vi "String Parser.vi"() -> ()   [LabVIEW 2017]
uses:
  <vilib>/regexp/Match Regular Expression.xnode
panel:
  out "String":string
  out "Array":T1(array[cluster])
  out "text":string
  in  "Path":path
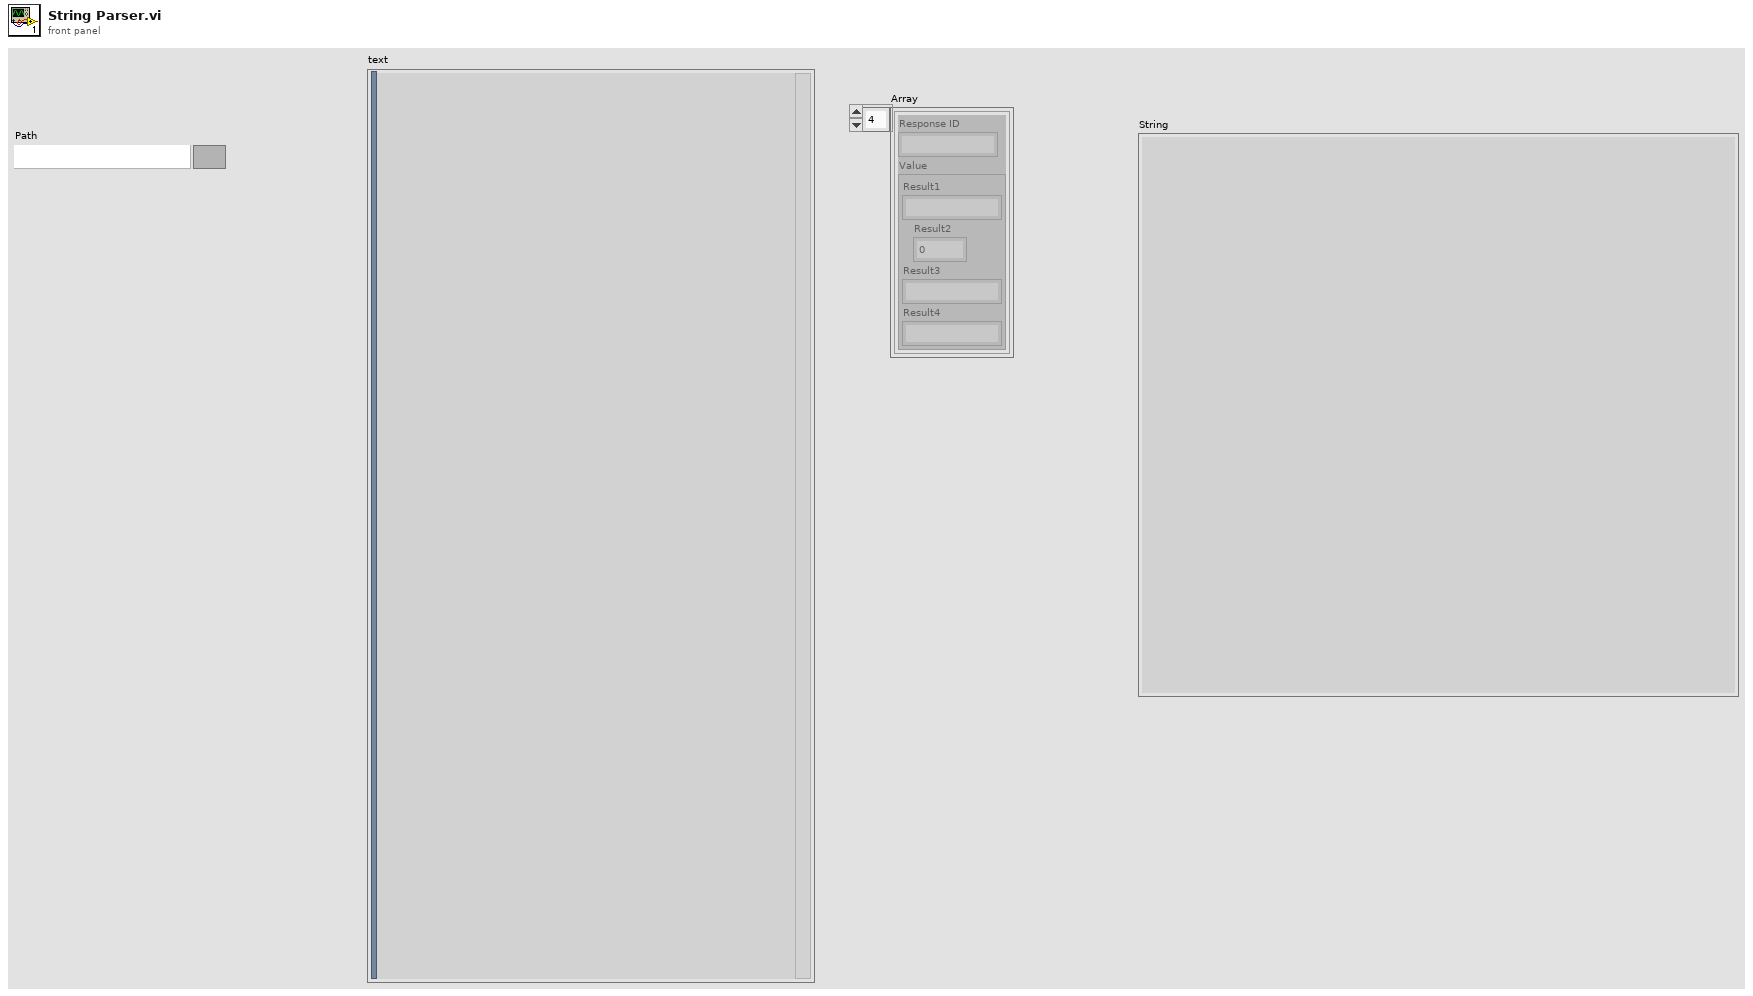
[diagram p1: front panel]
types:
  T1 = cluster{"Response ID":string, "Value":cluster{"Result1":string, "Result2":dbl, "Result3":string, "Result4":string}}[]
  T2 = cluster{"Response ID":string, "Value":cluster{"Result1":string, "Result2":dbl, "Result3":string, "Result4":string}}
  T3 = cluster{"Result1":string, "Result2":dbl, "Result3":string, "Result4":string}
  T4 = cluster{"Result1":string, "Result2":string, "Result3":string, "Result4":string}
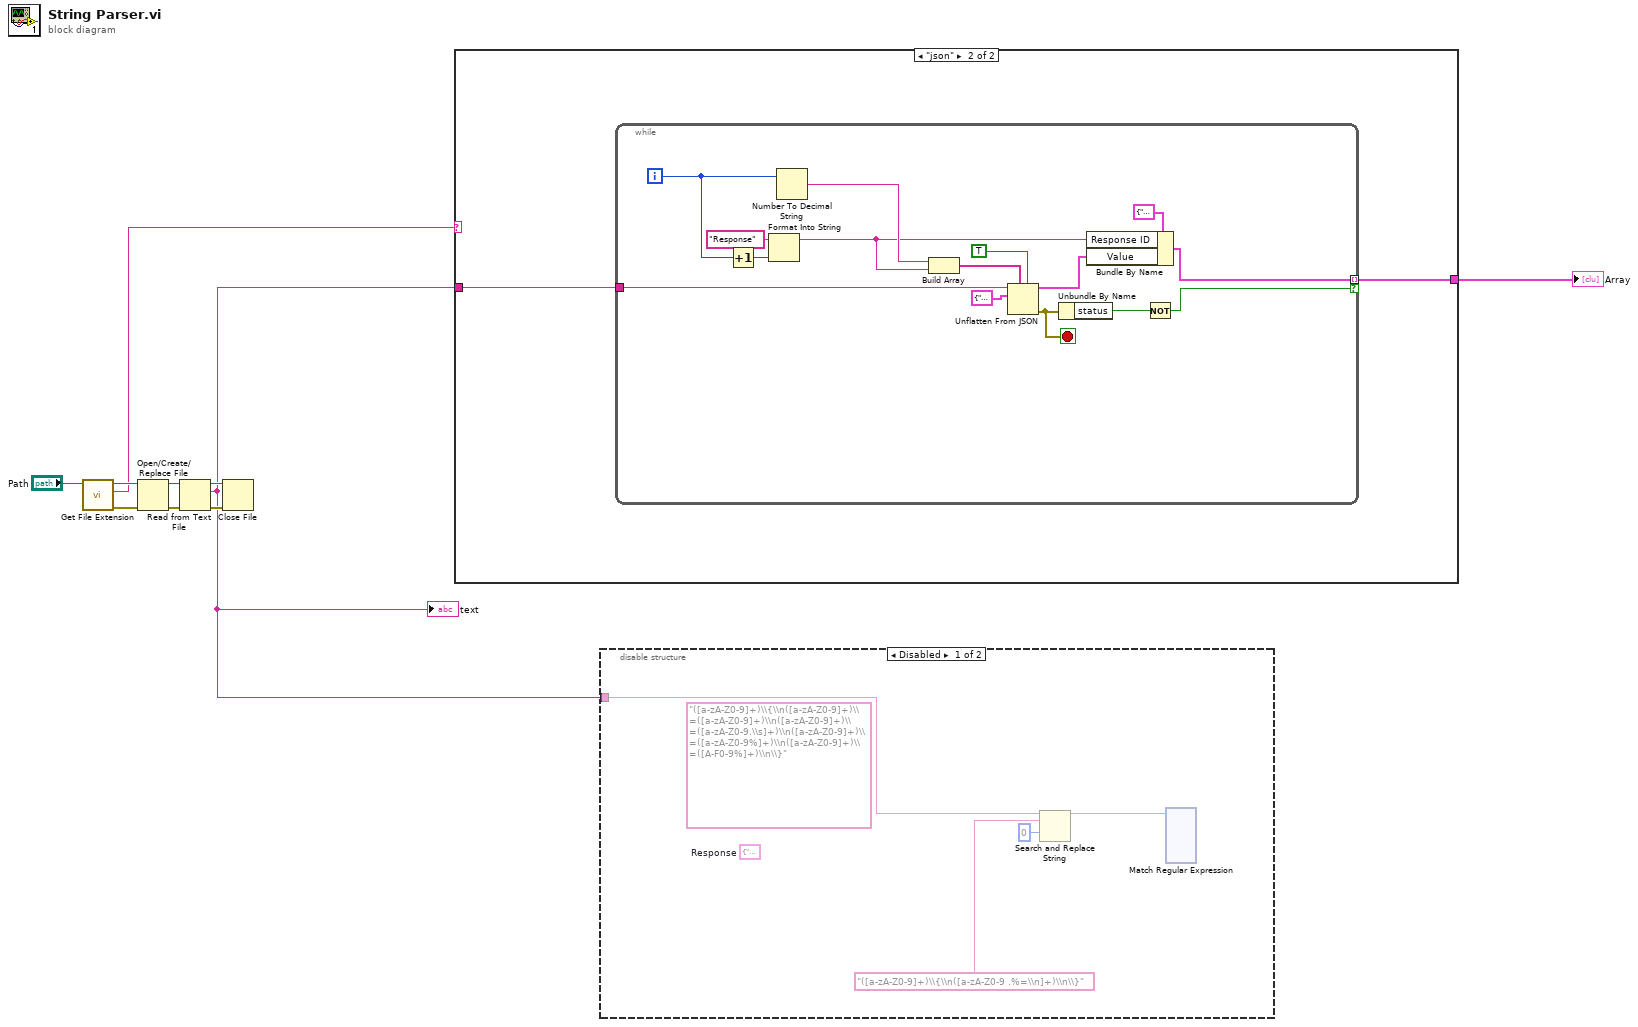
[diagram p0: block diagram]
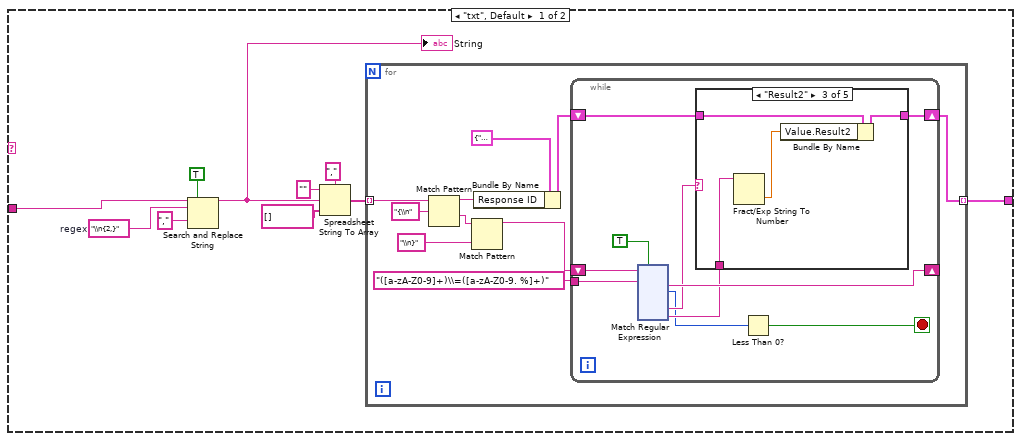
[diagram p2: hidden frame]
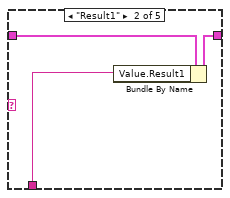
[diagram p4: hidden frame]
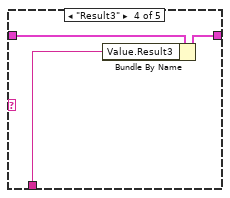
[diagram p5: hidden frame]
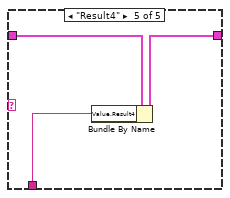
[diagram p6: hidden frame]
diagram:
  n1 = call <vilib>:"Get File Extension.vi"("file"="Path") -> ("error out"=w1:errorcluster, "lowercase file extension"=w4:string)  [unwired: 6 in, 3 out]
  n2 = Open/Create/Replace File(file path (use dialog)="Path", error in=w1) -> (refnum out=w9:refnum<file>, error out=w8:errorcluster)  [unwired: 4 in, 1 out]
  n3 = Read from Text File(file (use dialog)=w9, error in=w8) -> (refnum out=w7:refnum<file>, text=w2:string, error out=w6:errorcluster)  [unwired: 2 in, 1 out]
  "text" <- w2
  n4 = Close File(refnum=w7, error in=w6) -> ()  [unwired: 2 out]
  n5 = case shown="\"json\"" w4 {
    tunnel: w2 -> [w19 w172]
    tunnel: [w10 w171] -> w3
    frame "txt", Default {
      w18 = "\\n{2,}"  # regex
      n6 = Search and Replace String(replace all?=TRUE ("replace all? (F)"), input string=w19, search string=w18, replace string="," ("replace string (\"\")")) -> (result string=w12:string)  [unwired: 4 in, 3 out]
      "String" <- w12
      n7 = Spreadsheet String To Array(delimiter (Tab)=",", format string="", spreadsheet string=w12, array type (2D Dbl)=string[] [] ("spreadsheet string")) -> (array=w11:string[])
      n8 = for {
        tunnel: w11 -> [w29] mode=indexing
        tunnel: [w20] -> w10 mode=indexing
        n9 = Match Pattern(string=w29, regular expression="{\\n") -> (before substring=w27:string, after substring=w26:string)  [unwired: 1 in, 2 out]
        n10 = Match Pattern(string=w26, regular expression="\\n}") -> (before substring=w21:string)  [unwired: 1 in, 3 out]
        n11 = Bundle By Name(cluster=T2 {"Response ID"="", "Value"={"Result1"="", "Result2"=0.0, "Result3"="", "Result4"=""}}, "Response ID"=w27) -> (w23:T2)
        n12 = while {
          tunnel: "([a-zA-Z0-9]+)\\=([a-zA-Z0-9. %]+)" ("regular expression") -> [w38]
          shift-right: [w34] -> _
          shift-left: w21 -> [w37]
          shift-right: [w35] -> w20
          shift-left: w23 -> [w36]
          stop <- w30 stop-if-true
          n13 = xnode "Match Regular Expression"("input string"=w37, "regular expression"=w38, "ignore case? (F)"=TRUE) -> ("after match"=w34:string, "offset past match"=w31:i32, "submatch 1"=w33:string, "submatch 2"=w32:string)  [unwired: 3 in, 3 out]
          n14 = case shown="\"Result2\"" w33 {
            tunnel: w36 -> [w40 w43 w47 w50 w53]
            tunnel: [w40 w42 w46 w49 w52] -> w35
            tunnel: w32 -> [_ w41 w45 w48 w51]
            frame "False", Default {
            }
            frame "Result1" {
              n15 = Bundle By Name(cluster=w43, "Value.Result1"=w41) -> (w42:T2)
            }
            frame "Result2" {
              n16 = Fract/Exp String To Number(string=w45) -> (number=w44:dbl)  [unwired: 3 in, 1 out]
              n17 = Bundle By Name(cluster=w47, "Value.Result2"=w44) -> (w46:T2)
            }
            frame "Result3" {
              n18 = Bundle By Name(cluster=w50, "Value.Result3"=w48) -> (w49:T2)
            }
            frame "Result4" {
              n19 = Bundle By Name(cluster=w53, "Value.Result4"=w51) -> (w52:T2)
            }
          }
          n20 = Less Than 0?(x=w31) -> (x < 0?=w30:bool)
        }
      }
    }
    frame "json" {
      n21 = while {
        tunnel: w172 -> [w187]
        tunnel: [w180] -> w171 mode=indexing if=w182
        i -> [w178]
        stop <- w184 stop-if-true
        n22 = Increment(x=w178) -> (x+1=w174:i32)
        n23 = Format Into String(initial string="Response", w174) -> (resulting string=w175:string)  [unwired: 2 in, 1 out]
        n24 = Number To Decimal String(number=w178) -> (decimal integer string=w177:string)  [unwired: 1 in]
        n25 = Build Array(w177, w175) -> (w176:string[])
        n26 = Unflatten From JSON(path=w176, enable LabVIEW extensions? (T)=TRUE, JSON string=w187, type and defaults=T3 {"Result1"="", "Result2"=0.0, "Result3"="", "Result4"=""}) -> (value=w179:T3, error out=w184:errorcluster)  [unwired: 3 in]
        n27 = Unbundle By Name(w184) -> ("status"=w183:bool)
        n28 = Bundle By Name(cluster=T2 {"Response ID"="", "Value"={"Result1"="", "Result2"=0.0, "Result3"="", "Result4"=""}}, "Response ID"=w175, "Value"=w179) -> (w180:T2)
        n29 = Not(x=w183) -> (.not. x?=w182:bool)
      }
    }
  }
  "Array" <- w3
  n30 = disable-structure shown="Disabled" {
    disable-tunnel: w2 -> [w188 _]
    frame Disabled {
      (unwired) T4 {"Result1"="", "Result2"="", "Result3"="", "Result4"=""}  # Response
      (unwired) "([a-zA-Z0-9]+)\\{\\n([a-zA-Z0-9]+)\\=([a-zA-Z0-9]+)\\n([a-zA-Z0-9]+)\\=([a-zA-Z0-9.\\s]+)\\n([a-zA-Z0-9]+)\\=([a-zA-Z0-9%]+)\\n([a-zA-Z0-9]+)\\=([A-F0-9%]+)\\n\\}" ("regular expression")
      n31 = Search and Replace String(input string=w188, search string="([a-zA-Z0-9]+)\\{\\n([a-zA-Z0-9 .%=\\n]+)\\n\\}", offset=0 ("offset (0)")) -> (result string=w191:string)  [unwired: 5 in, 3 out]
      n32 = xnode "Match Regular Expression"("input string"=w191) -> ()  [unwired: 5 in, 7 out]
    }
    frame Enabled {
    }
  }
